vi "FGV_Queue Manager.vi"(7 "Methods":enum16{"Init", "Get", "Release", "Destroy"}(ring)=enum."Get", 8 "error in (no error)":errorcluster caption="错误输入（无错误）", 11 "Name":string) -> (0 "error out":errorcluster caption="错误输出", 2 "New?":bool, 3 "Queue":refnum<queue>)   [LabVIEW 2018, in "CAN FD.lvlib"]
uses:
  CAN FD.lvlib
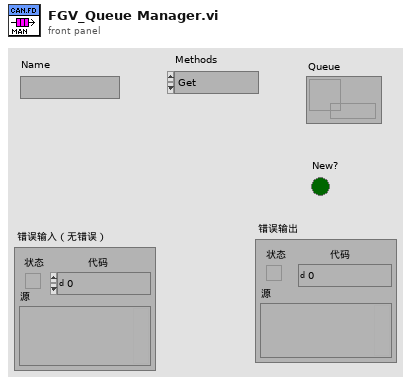
[diagram p1: front panel]
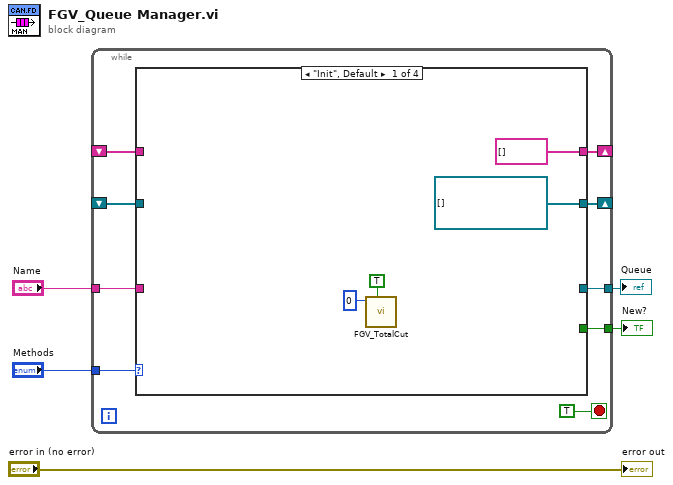
[diagram p0: block diagram]
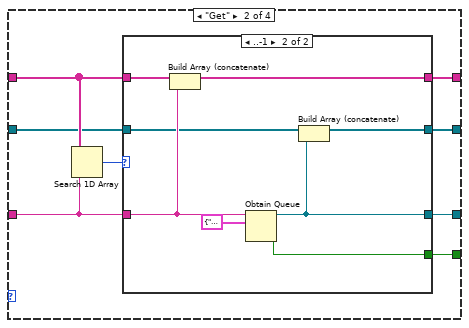
[diagram p2: hidden frame]
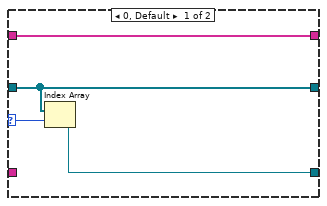
[diagram p3: hidden frame]
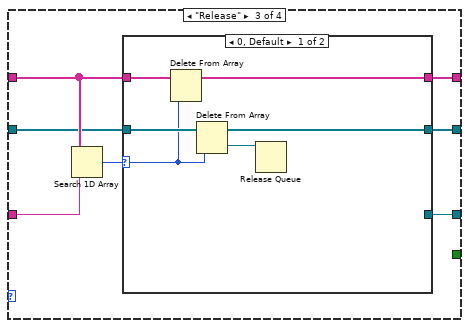
[diagram p4: hidden frame]
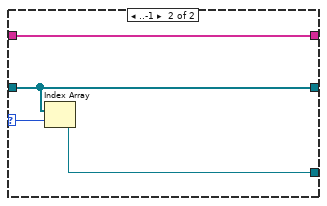
[diagram p5: hidden frame]
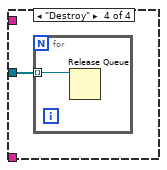
[diagram p6: hidden frame]
diagram:
  n1 = while {
    tunnel: "Methods" -> [w13]
    shift-right: [w12] -> _
    shift-left: _ -> [w11]
    shift-right: [w10] -> _
    shift-left: _ -> [w9]
    tunnel: "Name" -> [w8]
    tunnel: [w7] -> w3
    tunnel: [w6] -> w2
    stop <- TRUE stop-if-true
    n2 = case shown="\"Init\", Default" w13 {
      tunnel: [string[] [] w22 w41 _] -> w12
      tunnel: w11 -> [_ w25 w44 _]
      tunnel: [refnum<queue>[] [] w21 w40 _] -> w10
      tunnel: w9 -> [_ w24 w43 w56]
      tunnel: w8 -> [_ w23 w42 _]
      tunnel: [_ w20 w39 _] -> w7
      tunnel: [_ w19 _ _] -> w6
      frame "Init", Default {
        n3 = call "FGV_TotalCut.vi"("Set"=TRUE, "Total cut"=0 ("TotalCount")) -> ()  [unwired: 8 in, 2 out]
      }
      frame "Get" {
        n4 = Search 1D Array(1D array=w25, element=w23) -> (index of element=w26:i32)  [unwired: 1 in]
        n5 = case shown="..-1" w26 {
          selector: w26 -> [w29 _]
          tunnel: w25 -> [w30 w38]
          tunnel: w24 -> [w28 w34]
          tunnel: w23 -> [_ w35]
          tunnel: [w30 w37] -> w22
          tunnel: [w28 w33] -> w21
          tunnel: [w27 w32] -> w20
          tunnel: [_ w31] -> w19
          frame 0, Default {
            n6 = Index Array(array=w28, index=w29) -> (element=w27:refnum<queue>)
          }
          frame ..-1 {
            n7 = Build Array (concatenate)(w38, w35) -> (w37:string[])
            n8 = Obtain Queue(name (unnamed)=w35, element data type=cluster{"ID":string, "Data":variant} {"ID"="", "Data"=variant}) -> (queue out=w32:refnum<queue>, created new?=w31:bool)  [unwired: 3 in, 1 out]
            n9 = Build Array (concatenate)(w34, w32) -> (w33:refnum<queue>[])
          }
        }
      }
      frame "Release" {
        n10 = Search 1D Array(1D array=w44, element=w42) -> (index of element=w45:i32)  [unwired: 1 in]
        n11 = case shown="0, Default" w45 {
          selector: w45 -> [w46 w54]
          tunnel: w44 -> [w51 w55]
          tunnel: w43 -> [w49 w53]
          tunnel: [w50 w55] -> w41
          tunnel: [w48 w53] -> w40
          tunnel: [_ w52] -> w39
          frame 0, Default {
            n12 = Delete From Array(array=w51, index=w46) -> (array with subset deleted=w50:string[])  [unwired: 1 in, 1 out]
            n13 = Delete From Array(array=w49, index=w46) -> (deleted portion=w47:refnum<queue>, array with subset deleted=w48:refnum<queue>[])  [unwired: 1 in]
            n14 = Release Queue(queue=w47) -> ()  [unwired: 2 in, 3 out]
          }
          frame ..-1 {
            n15 = Index Array(array=w53, index=w54) -> (element=w52:refnum<queue>)
          }
        }
      }
      frame "Destroy" {
        n16 = for {
          tunnel: w56 -> [w57] mode=indexing
          n17 = Release Queue(queue=w57) -> ()  [unwired: 2 in, 3 out]
        }
      }
    }
  }
  "Queue" <- w3
  "New?" <- w2
  "error out" <- "error in (no error)"
